vi "Search for Subordinate.vi"(8 "error in":errorcluster, 10 "Identifier":string, 11 "Manual UI in":refnum<class "Manual UI.lvclass">) -> (0 "error out":errorcluster, 1 "Found":bool, 2 "Enqueuer":refnum<class "Message Enqueuer.lvclass">, 3 "Manual UI out":refnum<class "Manual UI.lvclass">, 4 "Index":i32)   [LabVIEW 2023, in "Manual UI.lvlib" / "Manual UI.lvclass"]
uses:
  Project/Manual UI.lvclass
  builds/Engine/Actor Framework.lvlibp/1abvi3w/vi.lib/ActorFramework/Message Enqueuer/Message Enqueuer.lvclass
  Project/Manual UI.lvclass/Manual UI.ctl
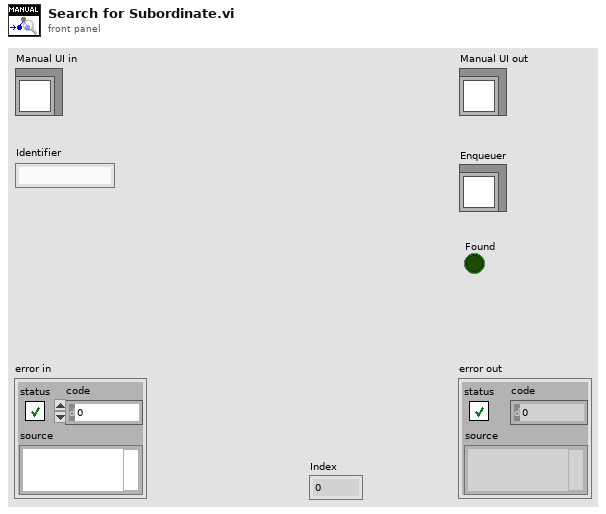
[diagram p1: front panel]
types:
  T1 = cluster{"Identifier":string, "Enqueuer":refnum<class "Message Enqueuer.lvclass">}[]
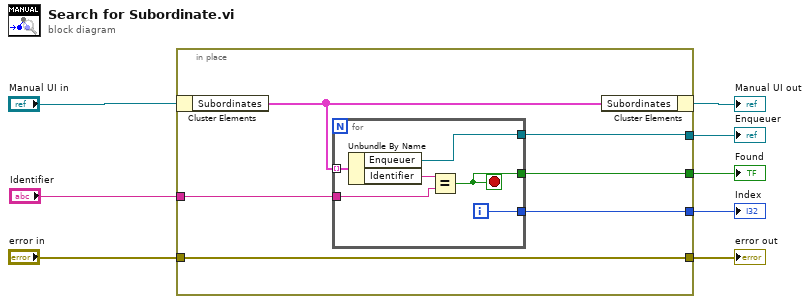
[diagram p0: block diagram]
diagram:
  n1 = in-place {
    in-place-border: [w14] -> w7
    in-place-border: "Identifier" -> [w12]
    in-place-border: "error in" -> [w11]
    in-place-border: [w11] -> w3
    in-place-border: [w10] -> w2
    in-place-border: [w9] -> w1
    n2 = in-place-cluster #1("Manual UI in") -> ("Subordinates"=w13:T1)
    n3 = for {
      tunnel: w13 -> [w20] mode=indexing
      tunnel: w12 -> [w18]
      tunnel: [w17] -> w10
      tunnel: [w16] -> w9
      tunnel: [w15] -> w14
      i -> [w16]
      stop <- w17 stop-if-true
      n4 = Unbundle By Name(w20) -> ("Enqueuer"=w15:refnum<class "Message Enqueuer.lvclass">, "Identifier"=w19:string)
      n5 = Equal?(x=w19, y=w18) -> (x = y?=w17:bool)
    }
    n6 = in-place-cluster #1("Subordinates"=w13) -> (→"Manual UI out":refnum<class "Manual UI.lvclass">)
  }
  "error out" <- w3
  "Enqueuer" <- w7
  "Found" <- w2
  "Index" <- w1
